vi "DHE_SetTiming.vi"(1 "num of Y amps":u16=1, 3 "num of X amps":u16=1, 4 "yroi start":i32, 5 "roi rows":i32, 6 "Num of amps":u32=1, 7 "roi cols":i32, 8 "error in":errorcluster, 9 "totysize":i32, 10 "totxsize":i32, 11 "Database RefNum out":T1) -> (0 "errorout":errorcluster, 2 "DET_READ_TIME":sgl=3.5 format="%.2f")   [LabVIEW 2016]
uses:
  DBSHAND/private/vis/DatabaseHand_RefNum.ctl
  DBSHAND/private/vis/DatabaseHand_Element_Set(U16).vi
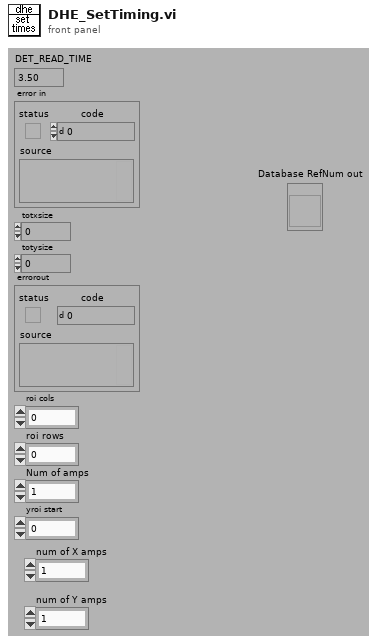
[diagram p1: front panel]
types:
  T1 = typedef "DatabaseHand_RefNum.ctl" = refnum<vi>
  T2 = typedef "CMN_TimingInfo.ctl" = cluster{"PixelTime":sgl, "SkipPixel":sgl, "SkipRow":sgl, "ShiftRow":sgl, "ShiftedPix":u16, "known_overhead":sgl, "DET_READ_TIME":sgl}
  T3 = enum16{"get fd", "set fd", "add ", "set_readtime", "get all", "clean all", "get by fd"}
  T4 = enum16{"get fd", "set fd", "add ", "set_readtime"}
  T5 = typedef "DHE_Device.ctl" = cluster{"DevNo":i32, "fd":i32, "name":string, "FPA":string, "modifiers":string, "binpatt":string, "readtime":dbl, "readmode":string, "type":string, "params":string}
  T6 = cluster{"Total Pixel read time":dbl, "Total serial skip time":dbl, "Total Paralel skip time":dbl, "Total Paralel shift time":dbl, "Total Read Time":dbl}
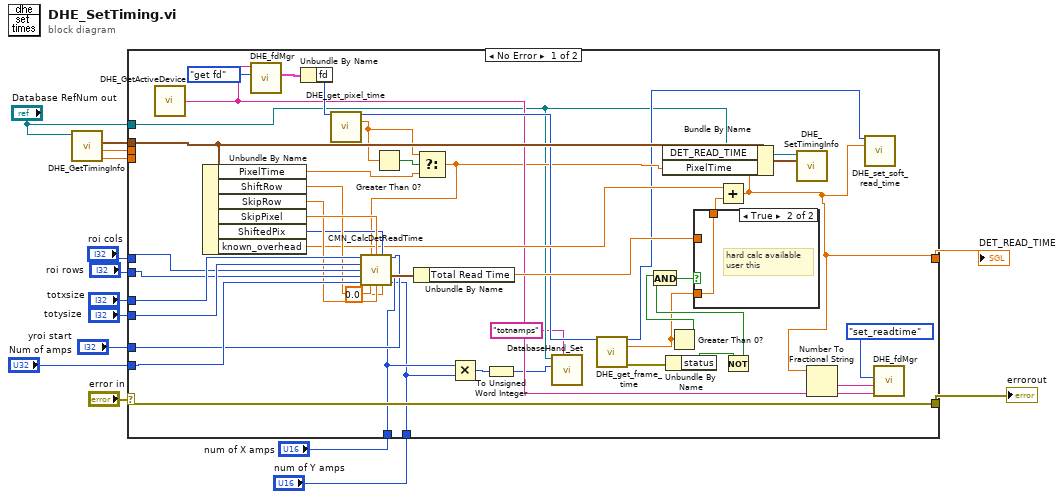
[diagram p0: block diagram]
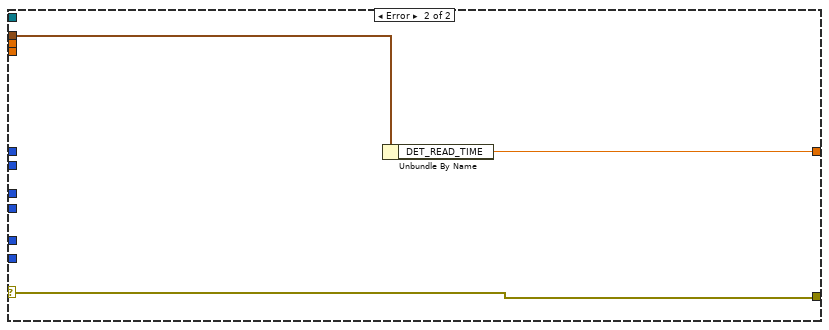
[diagram p3: hidden frame]
diagram:
  n1 = call "DHE_GetTimingInfo.vi"("Database RefNum out"="Database RefNum out") -> ("exposure_overhead"=w1:dbl, "seqs_overhead"=w2:dbl, "Timing"=w11:T2)  [unwired: 8 out]
  n2 = case shown="No Error" "error in" {
    selector: "error in" -> [w57 w63]
    tunnel: "totxsize" -> [w55 _]
    tunnel: "totysize" -> [w54 _]
    tunnel: [w57 w63] -> w12
    tunnel: w11 -> [w56 w62]
    tunnel: [w23 w61] -> w10
    tunnel: "roi cols" -> [w53 _]
    tunnel: "roi rows" -> [w52 _]
    tunnel: "Num of amps" -> [w51 _]
    tunnel: "Database RefNum out" -> [w21 _]
    tunnel: "yroi start" -> [w45 _]
    tunnel: "num of X amps" -> [w20 _]
    tunnel: "num of Y amps" -> [w19 _]
    tunnel: w2 -> [_ _]
    tunnel: w1 -> [_ _]
    frame No Error {
      n3 = call "DHE_GetActiveDevice.vi"() -> ("DHE_ActiveDevice"=w28:string)  [unwired: 9 out]
      n4 = Unbundle By Name(w56) -> ("PixelTime"=w25:sgl, "ShiftRow"=w49:sgl, "SkipRow"=w48:sgl, "SkipPixel"=w50:sgl, "ShiftedPix"=w47:u16, "known_overhead"=w32:sgl)
      n5 = call "DHE_fdMgr.vi"("action"=T3."get fd", "cmd in"=w28) -> ("Device"=w41:T5)  [unwired: 3 in, 6 out]
      n6 = Unbundle By Name(w41) -> ("fd"=w30:i32)
      n7 = call "DHE_get_pixel_time.vi"("fd in"=w30) -> ("fd out"=w29:i32, "pix_time (usecs)"=w26:sgl)  [unwired: 1 in, 12 out]
      n8 = Greater Than 0?(x=w26) -> (x > 0?=w27:bool)
      n9 = Select(t=w26, s=w27, f=w25) -> (s? t:f=w24:sgl)
      n10 = call "CMN_CalcDetReadTime.vi"("Det Columns"=w55, "Pixel Read Time (usecs)"=w24, "Serial Skip Time (usecs)"=w50, "skips_per_row_shift"=w47, "y roi start"=w45, "Det Rows"=w54, "cols"=w53, "rows"=w52, "num of X amps"=w20, "Num of amps"=w51, "Paralel Shift Time (usecs)"=w49, "Parallel Skip Time (usecs)"=w48, "overhead"=sgl 0.0 ("frame overhead"), "num of Y amps"=w19) -> ("Timing_out"=w46:T6)  [unwired: 1 out]
      n11 = Unbundle By Name(w46) -> ("Total Read Time"=w34:dbl)
      n12 = Multiply(x=w20, y=w19) -> (x*y=w17:u16)
      n13 = To Unsigned Word Integer(number=w17) -> (unsigned 16bit integer=w16:u16)
      n14 = call-poly "DatabaseHand_Set.vi"("name"="totnamps", "value"=w16, "Database RefNum in"=w21) -> ()  [unwired: 5 in, 4 out]
      n15 = call "DHE_get_frame_time.vi"("fd in"=w29) -> ("fd out"=w22:i32, "frame_time"=w35:dbl, "error out"=w40:errorcluster)  [unwired: 1 in, 11 out]
      n16 = Unbundle By Name(w40) -> ("status"=w39:bool)
      n17 = Greater Than 0?(x=w35) -> (x > 0?=w38:bool)
      n18 = Not(x=w39) -> (.not. x?=w37:bool)
      n19 = And(x=w38, y=w37) -> (x .and. y?=w36:bool)
      n20 = case shown="True" w36 {
        tunnel: w35 -> [_ w60]
        tunnel: [w59 w60] -> w33
        tunnel: w34 -> [w59 _]
        frame False {
          # "hard time not\nsupp. Use\nlocal estimation"
        }
        frame True {
          # "hard calc available\nuser this"
        }
      }
      n21 = Add(x=w32, y=w33) -> (x+y=w23:dbl)
      n22 = Bundle By Name(cluster=w56, "DET_READ_TIME"=w23, "PixelTime"=w24) -> (w58:T2)
      n23 = call "DHE_SetTimingInfo.vi"("Timing"=w58, "Database RefNum out"=w21) -> ()  [unwired: 10 out]
      n24 = Number To Fractional String(number=w23) -> (F-format string=w43:string)  [unwired: 3 out]
      n25 = call "DHE_set_soft_read_time.vi"("fd in"=w22, "readtime(secs)"=w23) -> ()  [unwired: 1 in, 13 out]
      n26 = call "DHE_fdMgr.vi"("arg in"=w43, "action"=T4."set_readtime", "cmd in"=w28) -> ()  [unwired: 2 in, 7 out]
    }
    frame Error {
      n27 = Unbundle By Name(w62) -> ("DET_READ_TIME"=w61:sgl)
    }
  }
  "errorout" <- w12
  "DET_READ_TIME" <- w10
